vi "ATSpectrograph_acceptCommand_homeLinearStage.vi"(8 "error in (no error)":errorcluster, 11 "command_homeLinearStage_Ctl":T1) -> (0 "error out":errorcluster, 2 "function return":i32, 3 "command_homeLinearStage_Ctl out":T1)   [LabVIEW 2016, in "SALLV_ATSpectrograph.lvlib"]
doc: "int ATSpectrograph_shm_acceptCommand_homeLinearStageLV(ATSpectrograph_command_homeLinearStageLV *command_homeLinearStage_Ctl );"
uses:
  SALLV_ATSpectrograph.lvlib
  DataTypes/command_homeLinearStage.ctl
  SALLV_ATSpectrograph.so
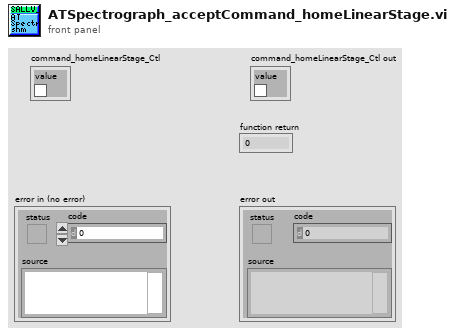
[diagram p1: front panel]
types:
  T1 = typedef "SALLV_ATSpectrograph.lvlib/command_homeLinearStage.ctl" = cluster{"value":bool}
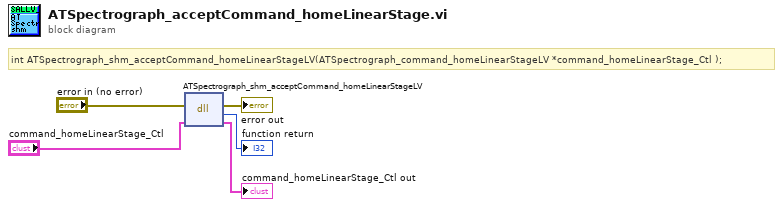
[diagram p0: block diagram]
diagram:
  # "int ATSpectrograph_shm_acceptCommand_homeLinearStageLV(ATSpectrograph_command_homeLinearStageLV *command_homeLinearStage_Ctl );"
  n1 = dll-call lib="home/harini/tcs/ts_AtSpectrograph/ts_sallv_AtSpectrograph/SALLV_ATSpectrograph.*" fn="ATSpectrograph_shm_acceptCommand_homeLinearStageLV"(error in="error in (no error)", "command_homeLinearStage_Ctl"="command_homeLinearStage_Ctl") -> (error out=→"error out":errorcluster, →"function return":i32, "command_homeLinearStage_Ctl"=→"command_homeLinearStage_Ctl out":T1)  [unwired: 2 in, 1 out]
